vi "add gating initalize(SubVI).vi"(9 "字符串":string, 10 "model":string="Delta") -> (0 "连接的字符串":string, 3 "ok or cancel":bool=TRUE)   [LabVIEW 2019, in "Add Seq.lvlib"]
uses:
  Add Seq.lvlib
  SubVI.lvlib
panel:
  in  "Compliance  Level (A)":dbl=0.0001
  in  "2400 resource name":refnum<visa-resource-name>
  out "错误输出":errorcluster
  in  "load":bool
  in  "cancel":bool
  in  "ok":bool
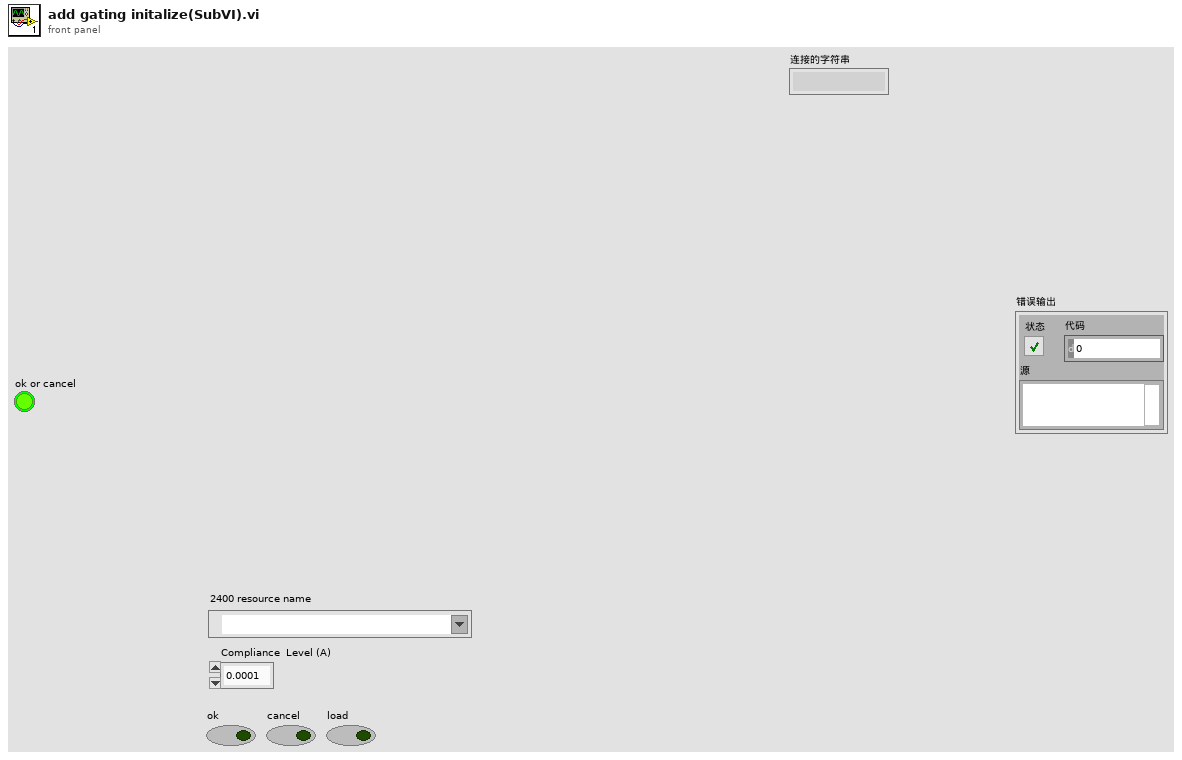
[diagram p1: front panel]
types:
  T1 = enum16{"open", "replace", "create", "open or create", "replace or create"}
  T2 = enum16{"open", "replace", "create", "open or create", "replace or create", "replace or create with confirmation"}
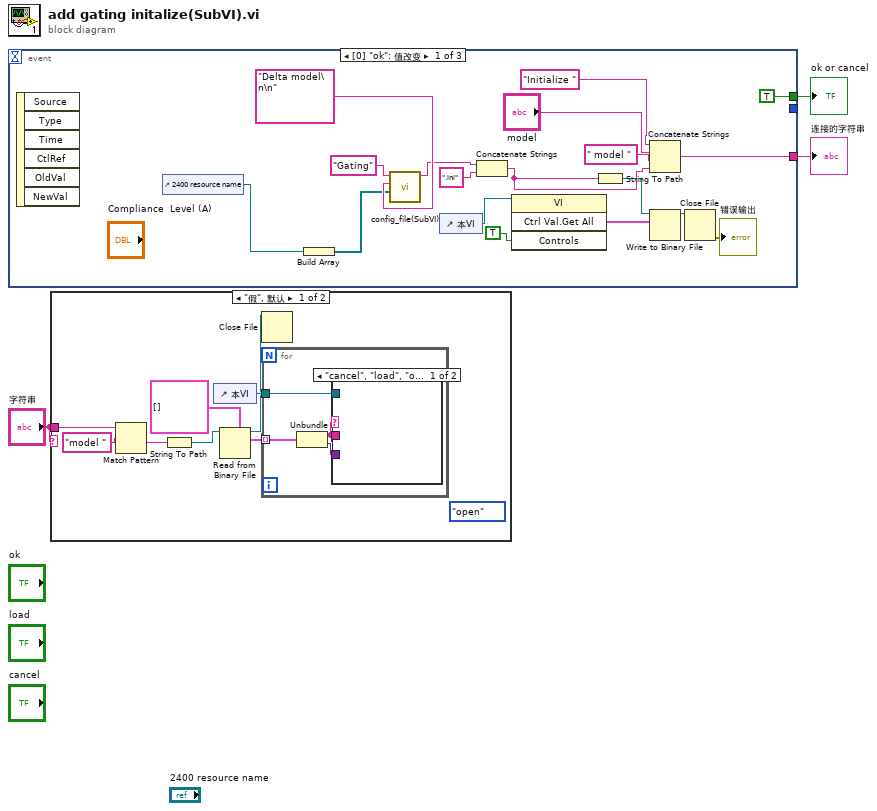
[diagram p0: block diagram]
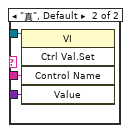
[diagram p2: hidden frame]
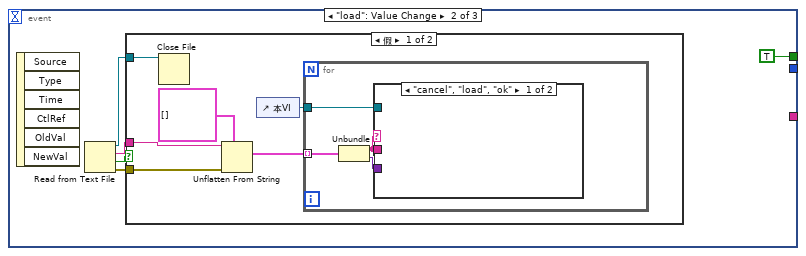
[diagram p4: hidden frame]
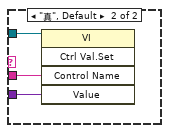
[diagram p5: hidden frame]
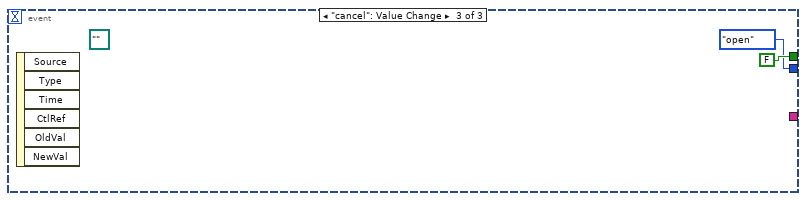
[diagram p7: hidden frame]
diagram:
  n1 = event shown="[0] \"ok\": 值改变" {
    selector: _ -> [_ _ _]
    dyn-events: _ -> [_ _ _]
    timeout: _ -> [_ _ _]
    tunnel: [_ _ T1."open" ("operation(0:open)")] -> _
    tunnel: [TRUE TRUE FALSE] -> w3
    tunnel: [w8 _ _] -> w2
    event "ok": Value Change {
      n2 = event-data() -> ()  [unwired: 1 in, 6 out]
      n3 = control-ref of="2400 resource name"() -> (w4:refnum<vi>)
      n4 = Build Array(w4) -> (w11:refnum<vi>[])
      n5 = call "config_file(SubVI).vi"("all ref"=w11, "文件抬头"="Delta model\n\n", "文件夹名称"="Gating" ("字符串")) -> ("字符串输出"=w15:string)  [unwired: 8 in]
      n6 = control-ref of="本VI"() -> (w18:refnum<vi>)
      n7 = Concatenate Strings(w15, ".ini" ("字符串")) -> (w13:string)
      n8 = invoke class="VI" method="Ctrl Val.Get All"(reference=w18, "Controls"=TRUE ("控件")) -> ("Get All Control Values Variant"=w6:cluster{"Name":string, "Variant Data":variant}[])  [unwired: 2 in, 3 out]
      n9 = String To Path(string=w13) -> (path=w7:path)
      n10 = Concatenate Strings("Initialize " ("字符串"), "model", " model " ("字符串"), w13) -> (w8:string)
      n11 = Write to Binary File(file (use dialog)=w7, data=w6) -> (refnum out=w5:refnum<file>)  [unwired: 4 in, 2 out]
      n12 = Close File(refnum=w5) -> (error out=→"错误输出":errorcluster)  [unwired: 1 in, 1 out]
    }
    event "load": Value Change {
      n13 = event-data() -> ()  [unwired: 1 in, 6 out]
      n14 = Read from Text File() -> (refnum out=w25:refnum<file>, text=w23:string, cancelled=w22:bool, error out=w24:errorcluster)  [unwired: 4 in]
      n15 = case shown="假" w22 {
        tunnel: w25 -> [w32 _]
        tunnel: w24 -> [w30 _]
        tunnel: w23 -> [w29 _]
        frame False {
          n16 = Close File(refnum=w32) -> ()  [unwired: 1 in, 2 out]
          n17 = Unflatten From String(type=cluster{"Name":string, "Variant Data":variant}[] [] ("控件值:获取全部"), binary string=w29, error in (no error)=w30) -> (value=w28:cluster{"Name":string, "Variant Data":variant}[])  [unwired: 2 in, 2 out]
          n18 = control-ref of="本VI"() -> (w27:refnum<vi>)
          n19 = for {
            tunnel: w28 -> [w36] mode=indexing
            tunnel: w27 -> [w35]
            n20 = Unbundle(w36) -> ("Name"=w33:string, "Variant Data"=w34:variant)
            n21 = case shown="\"cancel\", \"load\", \"ok\"" w33 {
              tunnel: w35 -> [_ w39]
              tunnel: w33 -> [_ w38]
              tunnel: w34 -> [_ w37]
              frame "cancel", "load", "ok" {
              }
              frame "真", Default {
                n22 = invoke class="VI" method="Ctrl Val.Set"(reference=w39, "Control Name"=w38, "Value"=w37) -> ()  [unwired: 2 in, 5 out]
              }
            }
          }
        }
        frame True {
        }
      }
    }
    event "cancel": Value Change {
      (unwired) path "" ("path")
      n23 = event-data() -> ()  [unwired: 1 in, 6 out]
    }
  }
  "ok or cancel" <- w3
  "连接的字符串" <- w2
  n24 = case shown="\"假\", 默认" "字符串" {
    tunnel: "字符串" -> [w49 _]
    frame "假", Default {
      (unwired) T2."open" ("操作(0:open)")
      n25 = Match Pattern(string=w49, regular expression="model " ("正则表达式")) -> (after substring=w48:string)  [unwired: 1 in, 3 out]
      n26 = String To Path(string=w48) -> (path=w45:path)
      n27 = control-ref of="本VI"() -> (w46:refnum<vi>)
      n28 = Read from Binary File(5:cluster{"Name":string, "Variant Data":variant}[] [] ("控件值:获取全部"), 11:w45) -> (2:w43:cluster{"Name":string, "Variant Data":variant}[], 3:w42:refnum<file>)  [unwired: 4 in, 2 out]
      n29 = Close File(refnum=w42) -> ()  [unwired: 1 in, 2 out]
      n30 = for {
        tunnel: w43 -> [w53] mode=indexing
        tunnel: w46 -> [w52]
        n31 = Unbundle(w53) -> ("Name"=w50:string, "Variant Data"=w51:variant)
        n32 = case shown="\"cancel\", \"load\", \"ok\"" w50 {
          tunnel: w52 -> [_ w56]
          tunnel: w50 -> [_ w55]
          tunnel: w51 -> [_ w54]
          frame "cancel", "load", "ok" {
          }
          frame "真", Default {
            n33 = invoke class="VI" method="Ctrl Val.Set"(reference=w56, "Control Name"=w55, "Value"=w54) -> ()  [unwired: 2 in, 5 out]
          }
        }
      }
    }
    frame "" {
    }
  }
